vi "Clear output buffer.vi"(8 "error in (no error)":errorcluster, 11 "VISA resource name":refnum<visa-resource-name>) -> (0 "error out":errorcluster, 3 "VISA resource name out":refnum<visa-resource-name>)   [LabVIEW 2012]
doc: "Clears the output buffer of the selected VISA resource by exhaustively reading it."
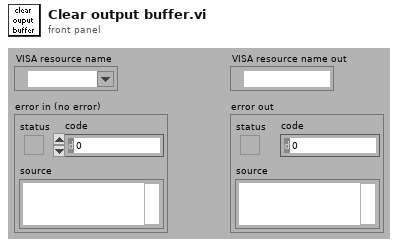
[diagram p1: front panel]
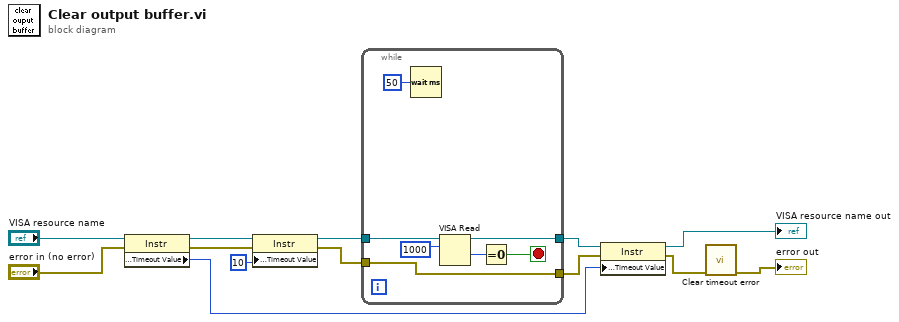
[diagram p0: block diagram]
diagram:
  n1 = property class="Instr"(reference="VISA resource name", error in="error in (no error)") -> (reference out=w11:refnum<visa-resource-name>, error out=w10:errorcluster, "General Settings:Timeout Value"=w4:u32)
  n2 = property class="Instr"(reference=w11, error in=w10, "General Settings:Timeout Value"=u32 10) -> (reference out=w8:refnum<visa-resource-name>, error out=w7:errorcluster)
  n3 = while {
    tunnel: w8 -> [w18]
    tunnel: w7 -> [w17]
    tunnel: [w17] -> w5
    tunnel: [w16] -> w6
    stop <- w19 stop-if-true
    n4 = Wait (ms)(milliseconds to wait=u32 50) -> ()  [unwired: 1 out]
    n5 = VISA Read(VISA resource name=w18, byte count=u32 1000) -> (VISA resource name out=w16:refnum<visa-resource-name>, return count=w20:u32)  [unwired: 1 in, 2 out]
    n6 = Equal To 0?(x=w20) -> (x = 0?=w19:bool)
  }
  n7 = property class="Instr"(reference=w6, error in=w5, "General Settings:Timeout Value"=w4) -> (reference out=→"VISA resource name out":refnum<visa-resource-name>, error out=w2:errorcluster)
  n8 = call "Clear timeout error.vi"("error in (no error)"=w2) -> ("error out"=→"error out":errorcluster)  [unwired: 10 out]
